vi "Test Returns Multiple Sections Added.vi"(11 "Test Case In":refnum<class "Diff Tool Test.lvclass">) -> (0 "error out":errorcluster, 3 "Test Case Out":refnum<class "Diff Tool Test.lvclass">)   [LabVIEW 2020, in "Diff Tool Test.lvclass"]
uses:
  Diff Tool Test.lvclass
panel:
  out "Result":string
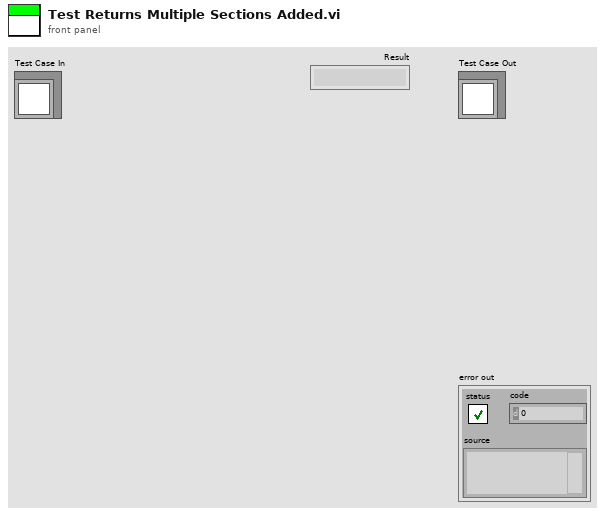
[diagram p1: front panel]
types:
  T1 = cluster{"Selection Start":u32, "Selection End":u32, "Type":enum16{"added", "missing"}}
  T2 = cluster{"Selection Start":u32, "Selection End":u32, "Type":enum16{"added", "missing"}}[]
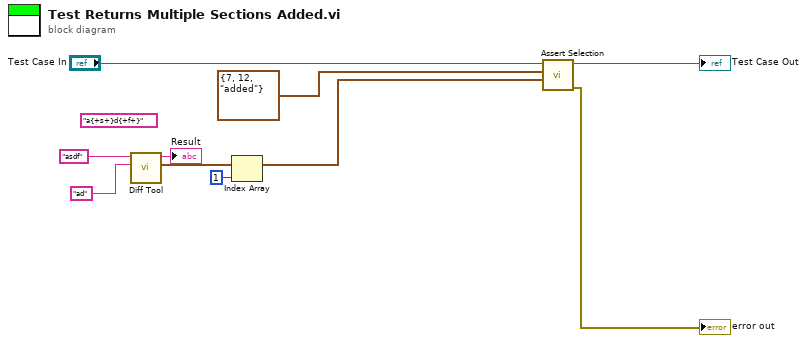
[diagram p0: block diagram]
diagram:
  (unwired) "a{+s+}d{+f+}" ("Reference")
  n1 = call "Diff Tool.vi"("Reference"="ad", "Target"="asdf") -> ("Highlights"=w5:T2, "Result"=→"Result":string)  [unwired: 8 in]
  n2 = Index Array(array=w5, index=1) -> (element=w4:T1)
  n3 = call "Assert Selection.vi"("Actual"=w4, "Expected"=T1 {"Selection Start"=7, "Selection End"=12, "Type"=enum."added"}, "Added Section Finder Test In"="Test Case In") -> ("error out"=→"error out":errorcluster, "Added Section Finder Test Out"=→"Test Case Out":refnum<class "Diff Tool Test.lvclass">)  [unwired: 7 in]
